vi "Host_Test.vi"() -> ()   [LabVIEW 2012]
uses:
  <vilib>/FPGAPlugInAG/PXIe-7962R/niLvFpga_Open_PXIe-7962R.vi
  <vilib>/rvi/interface/common/dynamic/niFpgaDynamicAddResources.vi
  <vilib>/Utility/error.llb/Error Cluster From Error Code.vi
  <vilib>/rvi/errors/niLvFpgaAdjustHostInterfaceError.vi
  <vilib>/FPGAPlugInAG/Dynamic/niLvFpga_Close_Dynamic.vi
  <vilib>/rvi/interface/nirviOpenFPGA/nirviOpenFPGA.xnode
  FPGA Bitfiles/AnalogIntegrator_NI5771_PXIe-7962R.lvbitx
  FPGA VIs/AnalogIntegrator_NI5771.vi
  <vilib>/rvi/interface/nirviReadWriteControl/nirviReadWriteControl.xnode
  <vilib>/rvi/interface/nirviMethod/nirviMethod.xnode
  <vilib>/rvi/interface/nirviCloseFPGA/nirviCloseFPGA.xnode
  NiFpgaLv.dll
  <vilib>/rvi/interface/Simulation/niFpgaSimulationCallBeginRW.vi
  <vilib>/FPGAPlugInAG/Dynamic/niLvFpga_ReadFifo_Dynamic.vi
  <vilib>/rvi/errors/niLvFpgaMergeErrorWithErrorCode.vi
panel:
  out "Samples per pixel":u32
  in  "Pixel time":dbl
  out "error out":errorcluster
  out "InterloopFIFO Overflow":bool
  out "ToHostCh1FIFO Overflow":bool
  out "Configured?":bool
  out "IO Module\\AI Over Range":bool
  out "Ch1":u32[](graph)
  # "microseconds"
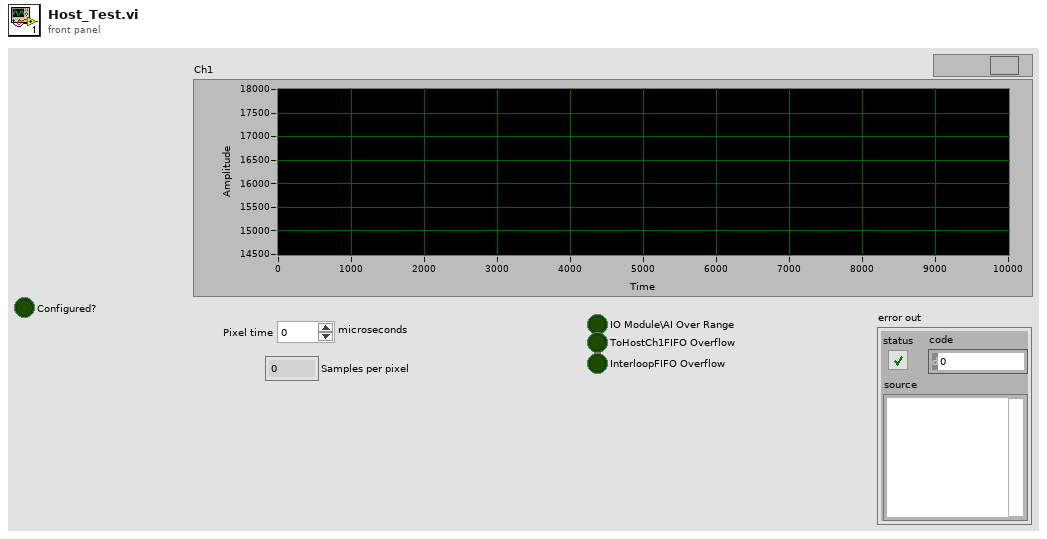
[diagram p1: front panel]
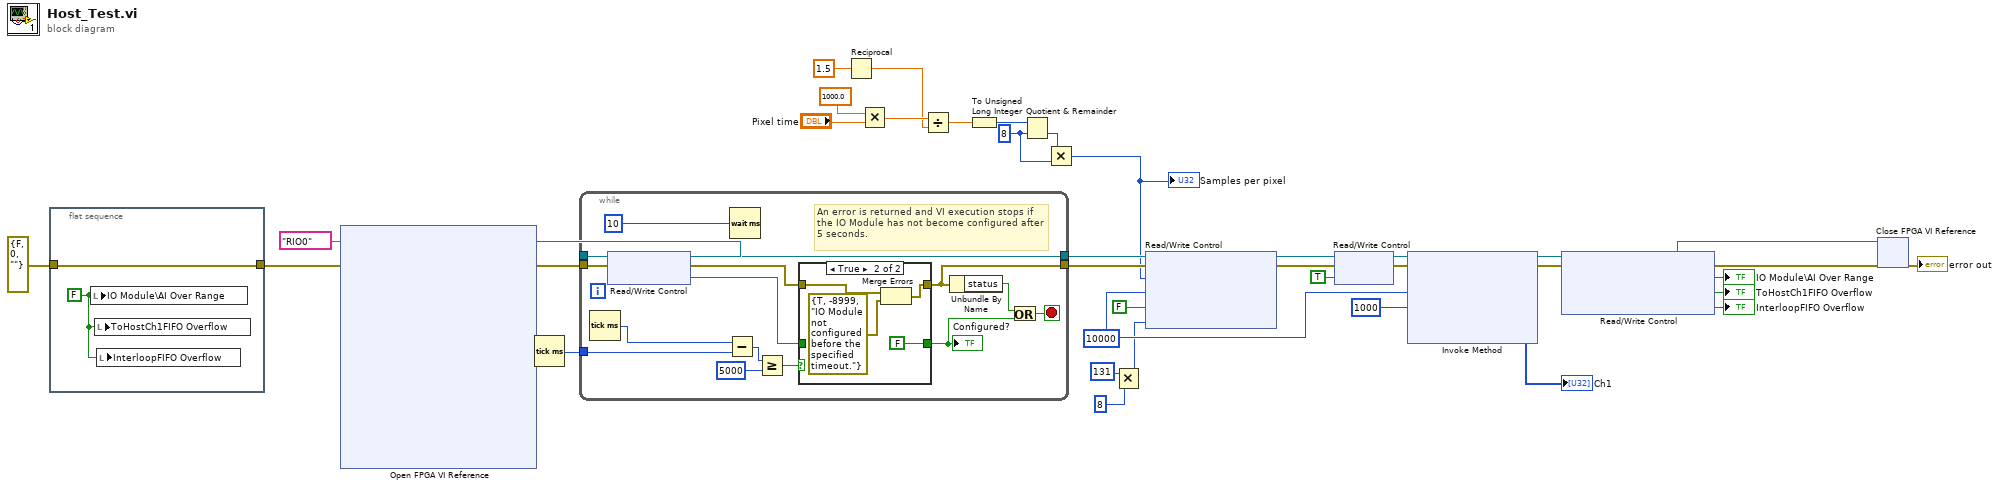
[diagram p0: block diagram]
diagram:
  w2 = u32 8 ("y")
  w29 = u32 10000 ("Requested pixels")
  n1 = flat-sequence {
    tunnel: errorcluster {"status"=FALSE, "code"=0, "source"=""} ("error in") -> [w39]
    tunnel: [w39] -> w12
    frame #0 {
      w40 = FALSE ("IO Module\\AI Over Range")
      n2 = local write "IO Module\\AI Over Range"(w40) -> ()
      n3 = local write "ToHostCh1FIFO Overflow"(w40) -> ()
      n4 = local write "InterloopFIFO Overflow"(w40) -> ()
    }
  }
  n5 = xnode "Open FPGA VI Reference"("error in"=w12, "resource name"=tag "RIO0") -> ("FPGA VI Reference Out"=w22:refnum<k20>, "error out"=w23:errorcluster)
  n6 = Tick Count (ms)() -> (millisecond timer value=w21:u32)
  n7 = while {
    tunnel: w23 -> [w48]
    tunnel: [w52] -> w20
    tunnel: [w44] -> w19
    tunnel: w22 -> [w47]
    tunnel: w21 -> [w42]
    stop <- w50 stop-if-true
    # "An error is returned and VI execution stops if the IO Module has not become configured after 5 seconds."
    n8 = Tick Count (ms)() -> (millisecond timer value=w43:u32)
    n9 = xnode "Read/Write Control"("FPGA VI Reference In"=w47, "error in"=w48) -> ("FPGA VI Reference Out"=w44:refnum<k20>, "error out"=w45:errorcluster, "Configured?"=w46:bool)
    n10 = Subtract(x=w43, y=w42) -> (x-y=w41:u32)
    n11 = Wait (ms)(milliseconds to wait=u32 10) -> ()  [unwired: 1 out]
    n12 = Greater Or Equal?(x=w41, y=u32 5000) -> (x >= y?=w53:bool)
    n13 = case shown="True" w53 {
      tunnel: [w57 FALSE ("Configured?")] -> w49
      tunnel: w46 -> [w57 _]
      tunnel: [w56 w60] -> w52
      tunnel: w45 -> [w56 w58]
      frame False {
      }
      frame True {
        n14 = Merge Errors(w58, errorcluster {"status"=TRUE, "code"=-8999, "source"="IO Module not configured before the specified timeout."} ("error in")) -> (w60:errorcluster)
      }
    }
    "Configured?" <- w49
    n15 = Unbundle By Name(w52) -> ("status"=w51:bool)
    n16 = Or(x=w51, y=w49) -> (x .or. y?=w50:bool)
  }
  n17 = Reciprocal(x=1.5) -> (1/x=w6:dbl)
  n18 = Multiply(x=1000.0, y="Pixel time") -> (x*y=w7:dbl)
  n19 = Divide(x=w7, y=w6) -> (x/y=w5:dbl)
  n20 = To Unsigned Long Integer(number=w5) -> (unsigned 32bit integer=w4:u32)
  n21 = Quotient & Remainder(x=w4, y=w2) -> (floor(x/y)=w3:u32)  [unwired: 1 out]
  n22 = Multiply(x=w3, y=w2) -> (x*y=w1:u32)
  "Samples per pixel" <- w1
  n23 = Multiply(x=131, y=8) -> (x*y=w16:i32)
  n24 = xnode "Read/Write Control"("FPGA VI Reference In"=w19, "error in"=w20, "Samples per pixel"=w1, "Requested pixels"=w29, "Acquire continuously"=FALSE, "Baselinex8 Ch1"=w16) -> ("FPGA VI Reference Out"=w35:refnum<k20>, "error out"=w36:errorcluster)
  n25 = xnode "Read/Write Control"("FPGA VI Reference In"=w35, "error in"=w36, "Acquire"=TRUE) -> ("FPGA VI Reference Out"=w33:refnum<k20>, "error out"=w32:errorcluster)
  n26 = xnode "Invoke Method"("FPGA VI Reference In"=w33, "error in"=w32, "Number of Elements"=w29, "Timeout (ms)"=1000) -> ("FPGA VI Reference Out"=w28:refnum<k20>, "error out"=w26:errorcluster, "Data"=→"Ch1":u32[])  [unwired: 1 out]
  n27 = xnode "Read/Write Control"("FPGA VI Reference In"=w28, "error in"=w26) -> ("FPGA VI Reference Out"=w27:refnum<k20>, "error out"=w25:errorcluster, "IO Module\\AI Over Range"=→"IO Module\\AI Over Range":bool, "ToHostCh1FIFO Overflow"=→"ToHostCh1FIFO Overflow":bool, "InterloopFIFO Overflow"=→"InterloopFIFO Overflow":bool)
  n28 = xnode "Close FPGA VI Reference"("FPGA VI Reference In"=w27, "error in"=w25) -> ("error out"=→"error out":errorcluster)
